vi "How often does string contain regular expression.vi"(3 "Regular expression":string, 4 "String":string) -> (14 "Number":i32)   [LabVIEW 2026]
doc: "This VI returns a count of the occurances of a regular expression in a string."
panel:
  # "This vi returns a count of the occurences of a regular expression in a string."
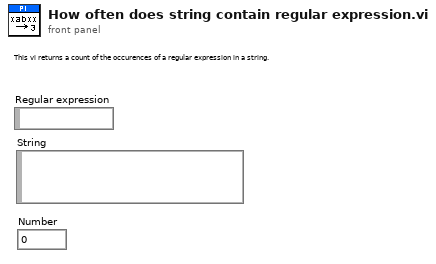
[diagram p1: front panel]
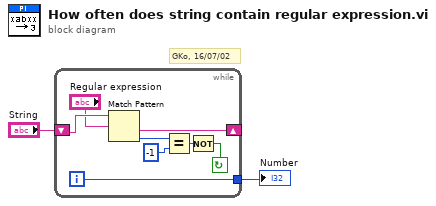
[diagram p0: block diagram]
diagram:
  # "GKo, 16/07/02"
  n1 = while {
    shift-left: "String" -> [w5]
    shift-right: [w4] -> _
    tunnel: [w7] -> w1
    i -> [w7]
    stop <- w6 continue-if-true
    n2 = Match Pattern(string=w5, regular expression="Regular expression") -> (after substring=w4:string, offset past match=w10:i32)  [unwired: 3 out]
    n3 = Equal?(x=w10, y=-1) -> (x = y?=w8:bool)
    n4 = Not(x=w8) -> (.not. x?=w6:bool)
  }
  "Number" <- w1
